vi "Page_AddStim.vi"(8 "error in (no error)":errorcluster, 11 "Configuration Paths":T1) -> (0 "error out":errorcluster, 3 "Configuration Paths out":T1)   [LabVIEW 2010]
uses:
  Config cluster.ctl
panel:
  in  "Delete":bool
  in  "Selected stimuls profiles (destination)":i32(listbox)
  in  "Add Stim":bool
  out "Procedure":string
  in  "Cancel Button":bool
  in  "OK Button":bool
  in  "Stimulus Profiles (source)":i32(listbox)
  # "1) Select your stimulus profile:"
  # "Available Stimuls Profiles"
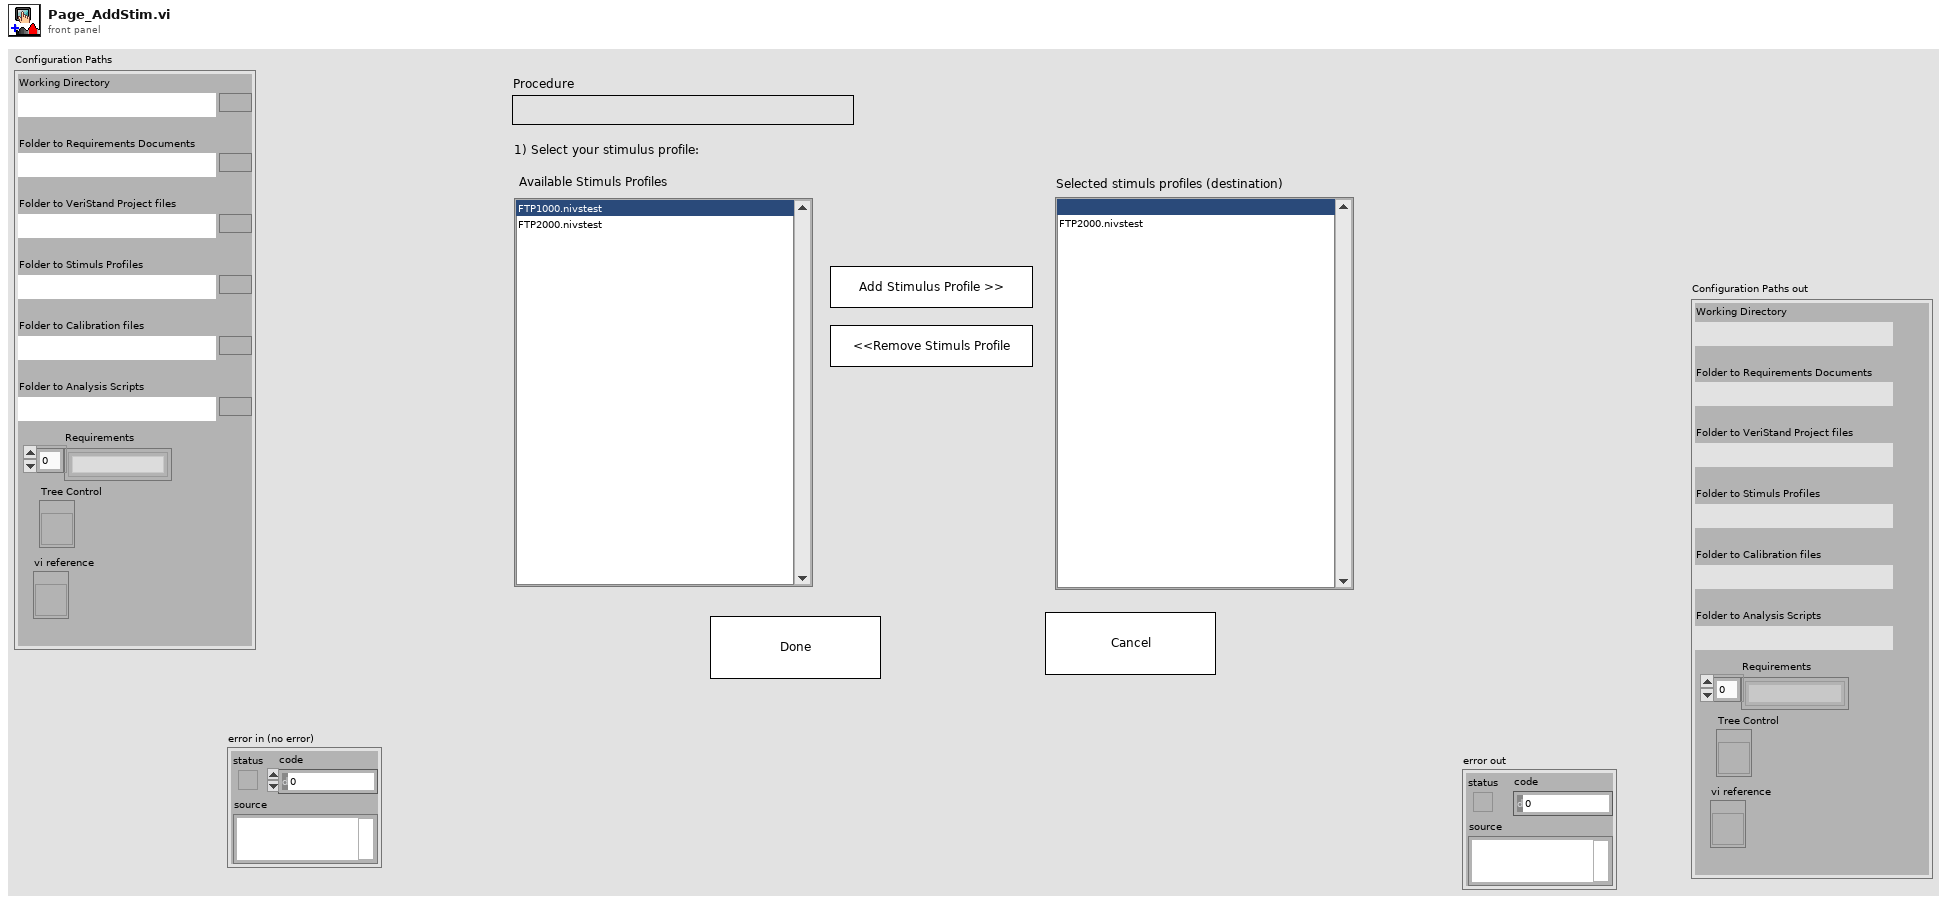
[diagram p1: front panel]
types:
  T1 = typedef "Config cluster.ctl" = cluster{"Working Directory":path, "Folder to Requirements Documents":path, "Folder to VeriStand Project files":path, "Folder to Stimuls Profiles":path, "Folder to Calibration files":path, "Folder to Analysis Scripts":path, "Requirements":string[], "Tree Control":refnum<vi>, "vi reference":refnum<vi>}
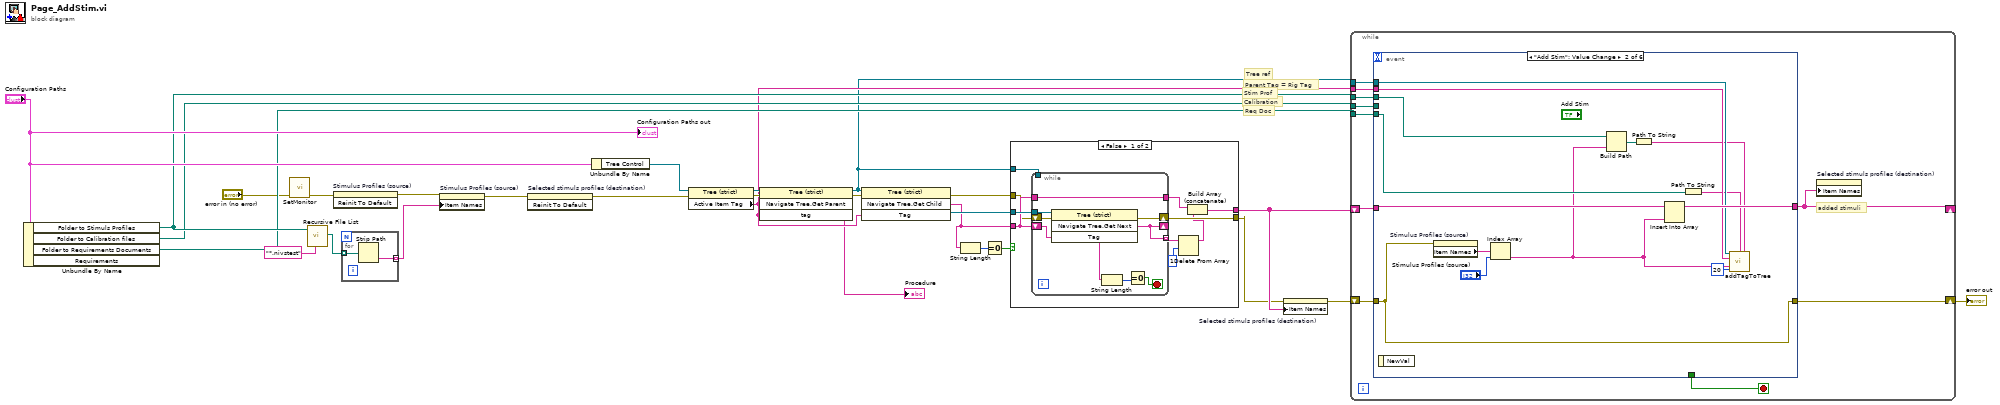
[diagram p0: block diagram]
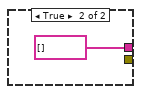
[diagram p2: hidden frame]
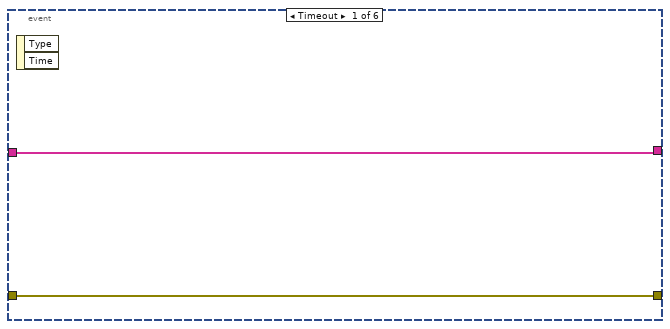
[diagram p3: hidden frame]
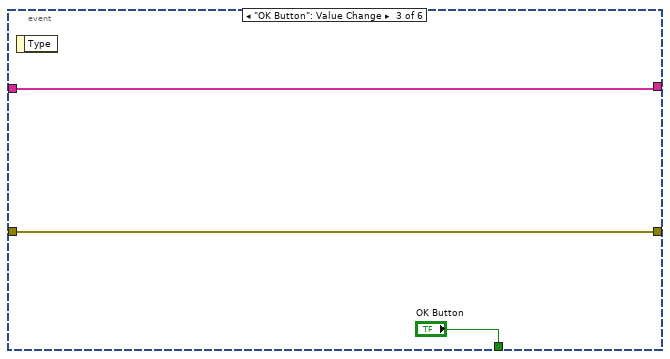
[diagram p4: hidden frame]
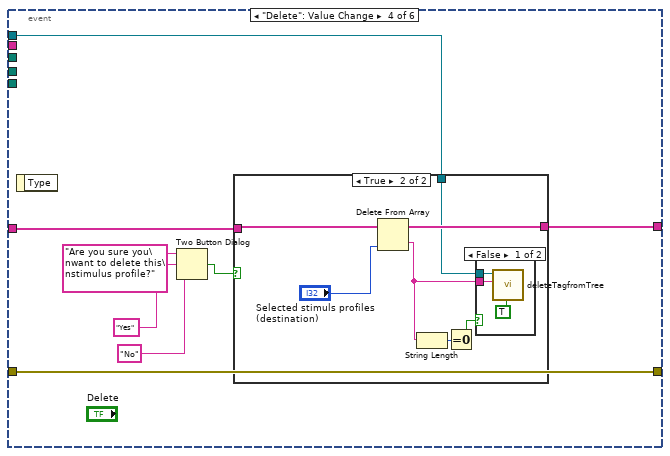
[diagram p5: hidden frame]
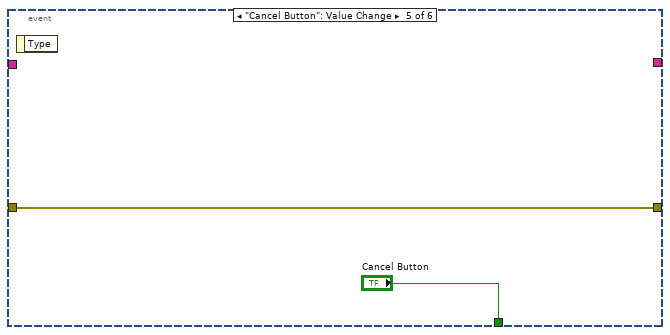
[diagram p8: hidden frame]
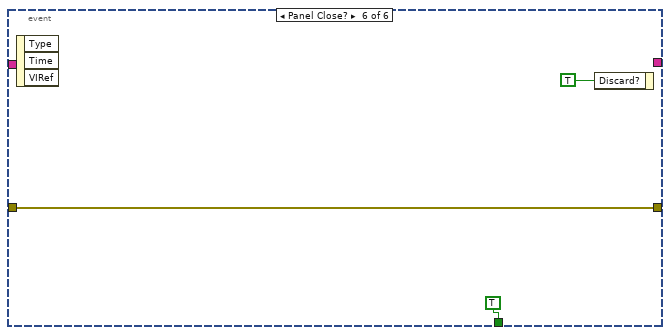
[diagram p9: hidden frame]
diagram:
  # "Req Doc"
  # "Calibration"
  # "Stim Prof"
  # "Parent Tag = Rig Tag"
  # "Tree ref"
  n1 = Unbundle By Name("Configuration Paths") -> ("Folder to Stimuls Profiles"=w14:path, "Folder to Calibration files"=w13:path, "Folder to Requirements Documents"=w12:path)  [unwired: 1 out]
  n2 = call "SetMonitor.vi"("error in (no error)"="error in (no error)") -> ("error out"=w2:errorcluster)  [unwired: 9 in, 1 out]
  n3 = call <vilib>:"Recursive File List.vi"("pattern"="*.nivstest", "Folder Path"=w14) -> ("All Files in Dir"=w23:path[])  [unwired: 5 in, 4 out]
  n4 = invoke on="Stimulus Profiles (source)" class="LstBox (strict)" method="Reinit To Default"(error in=w2) -> (error out=w16:errorcluster)  [unwired: 2 in, 2 out]
  n5 = for {
    tunnel: w23 -> [w30] mode=indexing
    tunnel: [w29] -> w22 mode=indexing
    n6 = Strip Path(path=w30) -> (name=w29:string)  [unwired: 1 out]
  }
  n7 = property on="Stimulus Profiles (source)" class="LstBox (strict)"(error in=w16, "Item Names"=w22) -> (error out=w11:errorcluster)  [unwired: 1 in, 1 out]
  n8 = invoke on="Selected stimuls profiles (destination)" class="LstBox (strict)" method="Reinit To Default"(error in=w11) -> (error out=w3:errorcluster)  [unwired: 2 in, 2 out]
  n9 = Unbundle By Name("Configuration Paths") -> ("Tree Control"=w17:refnum<vi>)
  n10 = property class="Tree (strict)"(reference=w17, error in=w3) -> (reference out=w10:refnum<vi>, error out=w9:errorcluster, "Active Item Tag"=w8:string)
  n11 = invoke class="Tree (strict)" method="Navigate Tree.Get Parent"(reference=w10, error in=w9, "tag"=w8) -> (reference out=w7:refnum<vi>, error out=w6:errorcluster, "Navigate Tree:Get Parent"=→"Procedure":string)  [unwired: 1 in, 1 out]
  n12 = invoke on="Invoke Node" class="Tree (strict)" method="Navigate Tree.Get Child"(reference=w7, error in=w6, "Tag"=w8) -> (reference out=w28:refnum<vi>, error out=w21:errorcluster, "Navigate Tree:Get Child"=w27:string)  [unwired: 1 in, 1 out]
  n13 = String Length(string=w27) -> (length=w26:i32)
  n14 = Equal To 0?(x=w26) -> (x = 0?=w25:bool)
  n15 = case shown="False" w25 {
    tunnel: [w40 _] -> w20
    tunnel: w7 -> [w39 _]
    tunnel: w28 -> [w38 _]
    tunnel: [w35 string[] []] -> w24
    tunnel: w27 -> [w36 _]
    tunnel: w21 -> [w34 _]
    frame False {
      n16 = while {
        tunnel: w39 -> [_]
        shift-right: [w45] -> _
        shift-left: w36 -> [w44]
        tunnel: [w45] -> w33 mode=indexing
        tunnel: w38 -> [w43]
        tunnel: [w42] -> w37
        tunnel: w36 -> [w42]
        shift-right: [w46] -> w40
        shift-left: w34 -> [w41]
        stop <- w47 stop-if-true
        n17 = invoke on="Invoke Node" class="Tree (strict)" method="Navigate Tree.Get Next"(reference=w43, error in=w41, "Tag"=w44) -> (error out=w46:errorcluster, "Navigate Tree:Get Next Item"=w45:string)  [unwired: 1 in, 2 out]
        n18 = String Length(string=w45) -> (length=w48:i32)
        n19 = Equal To 0?(x=w48) -> (x = 0?=w47:bool)
      }
      n20 = Delete From Array(array=w33, length=1) -> (array with subset deleted=w31:string[])  [unwired: 1 in, 1 out]
      n21 = Build Array (concatenate)(w37, w31) -> (w35:string[])
    }
    frame True {
    }
  }
  n22 = property on="Selected stimuls profiles (destination)" class="LstBox (strict)"(error in=w20, "Item Names"=w24) -> (error out=w19:errorcluster)  [unwired: 1 in, 1 out]
  n23 = while {
    shift-right: [w55] -> _
    shift-left: w24 -> [w56]
    tunnel: w7 -> [w54]
    tunnel: w8 -> [w53]
    shift-right: [w50] -> w18
    shift-left: w19 -> [w51]
    tunnel: w14 -> [w59]
    tunnel: w13 -> [w57]
    tunnel: w12 -> [w52]
    stop <- w58 stop-if-true
    # "added stimuli"
    n24 = event shown="[1] \"Add Stim\": Value Change" {
      selector: _ -> [_ _ _ _ _ _]
      dyn-events: _ -> [_ _ _ _ _ _]
      timeout: _ -> [_ _ _ _ _ _]
      tunnel: w59 -> [_ w65 _ _ _ _]
      tunnel: [_ _ "OK Button" _ "Cancel Button" TRUE ("Cancel Button")] -> w58
      tunnel: w57 -> [_ _ _ _ _ _]
      tunnel: w56 -> [w60 w75 w77 w86 _ _]
      tunnel: [w60 w74 w77 w85 _ _] -> w55
      tunnel: w54 -> [_ w71 _ w84 _ _]
      tunnel: w53 -> [_ w70 _ _ _ _]
      tunnel: w52 -> [_ w64 _ _ _ _]
      tunnel: w51 -> [w61 w62 w76 w79 w98 w102]
      tunnel: [w61 w62 w76 w79 w98 w102] -> w50
      event Timeout {
        n25 = event-data() -> ()  [unwired: 1 in, 2 out]
      }
      event "Add Stim": Value Change {
        n26 = event-data() -> ()  [unwired: 1 in, 1 out]
        n27 = property on="Stimulus Profiles (source)" class="LstBox (strict)"(error in=w62) -> ("Item Names"=w73:string[])  [unwired: 1 in, 2 out]
        n28 = Index Array(array=w73, index="Stimulus Profiles (source)") -> (element=w63:string)
        n29 = Build Path(base path=w65, name or relative path=w63) -> (appended path=w68:path)
        n30 = Path To String(path=w68) -> (string=w67:string)
        n31 = Insert Into Array(array=w75, new element=w63) -> (w74:string[])  [unwired: 1 in]
        n32 = Path To String(path=w64) -> (string=w66:string)
        n33 = call "addTagToTree.vi"("Tree ref"=w71, "Stimulus path"=w67, "parent tag"=w70, "new tag"=w63, "Symbol"=20, "Req doc path"=w66) -> ()  [unwired: 9 in, 1 out]
      }
      event "OK Button": Value Change {
        n34 = event-data() -> ()  [unwired: 1 in, 1 out]
      }
      event "Delete": Value Change {
        n35 = event-data() -> ()  [unwired: 1 in, 1 out]
        n36 = Two Button Dialog(message="Are you sure you\nwant to delete this\nstimulus profile?", 1:"No" ("F button name (\"Cancel\")"), 2:"Yes" ("T button name (\"OK\")")) -> (T button?=w80:bool)
        n37 = case shown="True" w80 {
          tunnel: w86 -> [w87 w93]
          tunnel: [w87 w92] -> w85
          tunnel: w84 -> [_ w91]
          frame False {
          }
          frame True {
            n38 = Delete From Array(array=w93, index="Selected stimuls profiles (destination)") -> (deleted portion=w90:string, array with subset deleted=w92:string[])  [unwired: 1 in]
            n39 = String Length(string=w90) -> (length=w89:i32)
            n40 = Equal To 0?(x=w89) -> (x = 0?=w88:bool)
            n41 = case shown="False" w88 {
              tunnel: w91 -> [w97 _]
              tunnel: w90 -> [w95 _]
              frame False {
                n42 = call "deleteTagfromTree.vi"("Delete Children?"=TRUE, "Tag"=w95, "Tree Ref"=w97) -> ()  [unwired: 7 in, 2 out]
              }
              frame True {
              }
            }
          }
        }
      }
      event "Cancel Button": Value Change {
        n43 = event-data() -> ()  [unwired: 1 in, 1 out]
      }
      event Panel Close? {
        n44 = event-data() -> ()  [unwired: 1 in, 3 out]
        n45 = event-data("Discard?"=TRUE) -> ()  [unwired: 1 in, 1 out]
      }
    }
    n46 = property on="Selected stimuls profiles (destination)" class="LstBox (strict)"("Item Names"=w55) -> ()  [unwired: 2 in, 2 out]
  }
  "error out" <- w18
  "Configuration Paths out" <- "Configuration Paths"
